vi "initial.vi"(8 "error in (no error)":errorcluster, 11 "Cell in":refnum<class "Cell.lvclass">) -> (0 "error out":errorcluster, 3 "Cell out":refnum<class "Cell.lvclass">)   [LabVIEW 2014, in "Cell.lvclass"]
uses:
  Cell.lvclass
  Cell.lvclass/Cell.ctl
panel:
  out "isCovered":bool
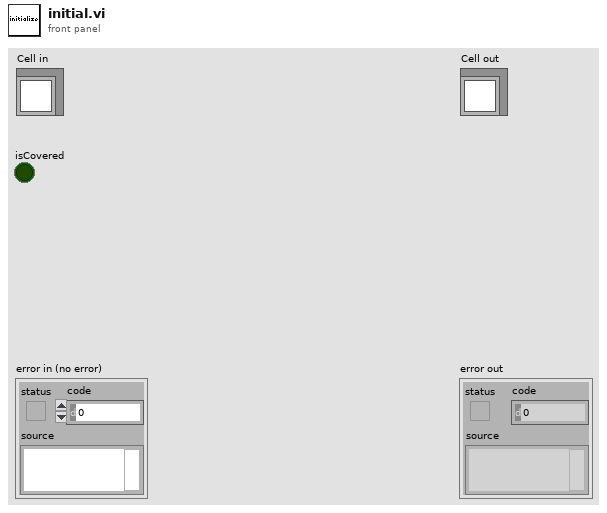
[diagram p1: front panel]
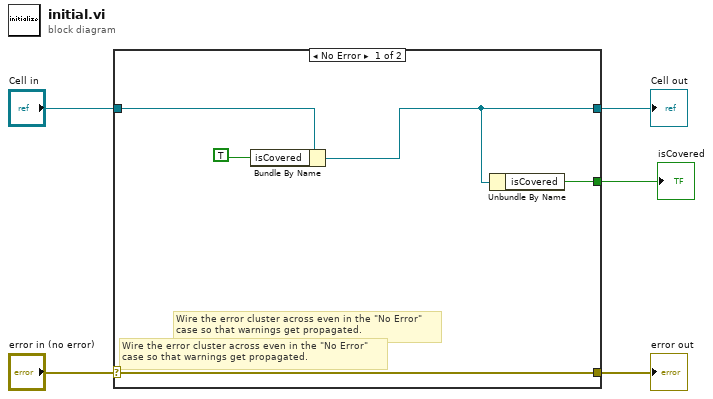
[diagram p0: block diagram]
diagram:
  n1 = case shown="No Error" "error in (no error)" {
    selector: "error in (no error)" -> [w10 w12]
    tunnel: [w10 w12] -> w4
    tunnel: [w8 w11] -> w1
    tunnel: "Cell in" -> [w9 w11]
    tunnel: [w7 _] -> w2
    frame No Error {
      # "Wire the error cluster across even in the \"No Error\"\ncase so that warnings get propagated."
      # "Wire the error cluster across even in the \"No Error\"\ncase so that warnings get propagated."
      n2 = Bundle By Name(cluster=w9, "isCovered"=TRUE) -> (w8:refnum<class "Cell.lvclass">)
      n3 = Unbundle By Name(w8) -> ("isCovered"=w7:bool)
    }
    frame Error {
    }
  }
  "error out" <- w4
  "Cell out" <- w1
  "isCovered" <- w2
